vi "ProcessSingleComic.vi"(8 "error in":errorcluster, 10 "Working Folder":path, 11 "Original Comic File":path) -> (0 "error out":errorcluster, 3 "Deleted files":string[](array[string]))   [LabVIEW 2022 SP3]
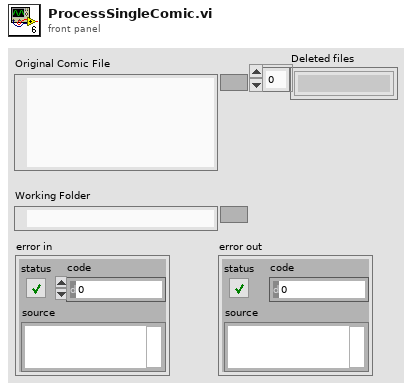
[diagram p1: front panel]
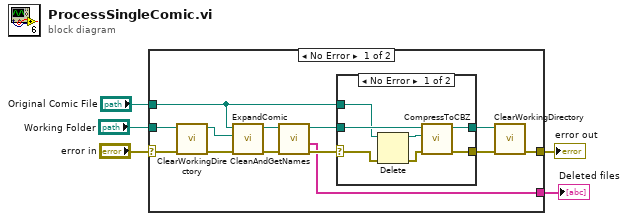
[diagram p0: block diagram]
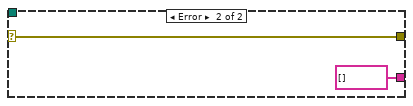
[diagram p3: hidden frame]
diagram:
  n1 = case shown="No Error" "error in" {
    selector: "error in" -> [w7 w29]
    tunnel: "Working Folder" -> [w18 _]
    tunnel: "Original Comic File" -> [w12 _]
    tunnel: [w9 w29] -> w3
    tunnel: [w6 string[] [] ("Deleted files")] -> w1
    frame No Error {
      n2 = call "ClearWorkingDirectory.vi"("error in"=w7, "Working Path"=w18) -> ("error out"=w17:errorcluster, "Working Path Out"=w16:path)  [unwired: 8 in]
      n3 = call "ExpandComic.vi"("error in (no error)"=w17, "Working Dir"=w16, "Source"=w12) -> ("error out"=w14:errorcluster, "Working Dir Out"=w15:path)  [unwired: 7 in]
      n4 = call "CleanAndGetNames.vi"("error in"=w14, "Working Dir"=w15) -> ("error out"=w13:errorcluster, "Deleted files"=w6:string[], "Working Dir Out"=w11:path)  [unwired: 6 in, 1 out]
      n5 = case shown="No Error" w13 {
        selector: w13 -> [w25 w27]
        tunnel: w12 -> [w22 _]
        tunnel: w11 -> [w24 w26]
        tunnel: [w20 w27] -> w10
        tunnel: [w19 w26] -> w8
        frame No Error {
          n6 = Delete(path (use dialog)=w22, error in=w25) -> (deleted path=w21:path, error out=w23:errorcluster)  [unwired: 3 in, 1 out]
          n7 = call "CompressToCBZ.vi"("error in"=w23, "FormerFilename"=w21, "Working Path"=w24) -> ("error out"=w20:errorcluster, "Working Path Out"=w19:path)  [unwired: 7 in]
        }
        frame Error {
        }
      }
      n8 = call "ClearWorkingDirectory.vi"("error in"=w10, "Working Path"=w8) -> ("error out"=w9:errorcluster)  [unwired: 8 in, 1 out]
    }
    frame Error {
    }
  }
  "error out" <- w3
  "Deleted files" <- w1
